vi "prediction.vi"(1 "X":dbl[][](array[numeric]), 2 "b":dbl, 3 "w":dbl[][](array[numeric])) -> (0 "Y_predicted":dbl[][](array[numeric]))   [LabVIEW 2020]
uses:
  <vilib>/Analysis/baseanly.llb/Real A x B.vi
  <vilib>/Analysis/Matrix/Numeric/Conversions/Array To Matrix - RA2.vi
  <vilib>/Analysis/Matrix/Numeric/Conversions/Matrix To Array - RM.vi
  <vilib>/Analysis/NI_AALBase.lvlib
  <vilib>/Analysis/Matrix/NI_Matrix.lvlib
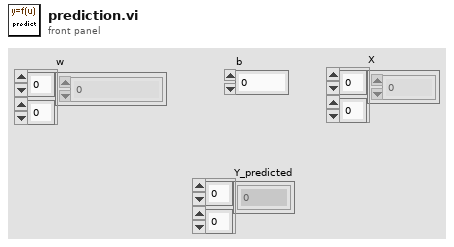
[diagram p1: front panel]
types:
  T1 = typedef "NI_Matrix.lvlib/RealMatrix.ctl" = dbl[][]
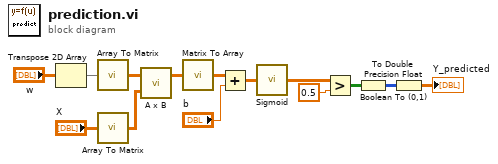
[diagram p0: block diagram]
diagram:
  n1 = Transpose 2D Array(2D array="w") -> (transposed array=w10:dbl[][])
  n2 = call-poly <vilib>:"Array To Matrix.vi"("Real 2D Array"=w10) -> ("Real Matrix"=w13:T1)
  n3 = call-poly <vilib>:"Array To Matrix.vi"("Real 2D Array"="X") -> ("Real Matrix"=w12:T1)
  n4 = call-poly <vilib>:"A x B.vi"("B"=w12, "A"=w13) -> ("A x B"=w14:T1)  [unwired: 1 out]
  n5 = call-poly <vilib>:"Matrix To Array.vi"("Real Matrix"=w14) -> ("Real 2D Array"=w8:dbl[][])
  n6 = Add(x=w8, y="b") -> (x+y=w7:dbl[][])
  n7 = call "Sigmoid.vi"("Z"=w7) -> ("Sigmoid(Z)"=w5:dbl[][])  [unwired: 2 in]
  n8 = Greater?(x=w5, y=0.5) -> (0:w3:bool[][])
  n9 = Boolean To (0,1)(Boolean=w3) -> (0, 1=w2:i16[][])
  n10 = To Double Precision Float(number=w2) -> (double precision float=→"Y_predicted":dbl[][])
